vi "Query Error.vi"(8 "error in (no error)":errorcluster, 11 "VISA resource name":refnum<visa-resource-name>) -> (0 "error out":errorcluster, 1 "Error Message":string, 2 "Error Code":i32[](array[numeric]), 3 "VISA resource name out":refnum<visa-resource-name>)   [LabVIEW 2023]
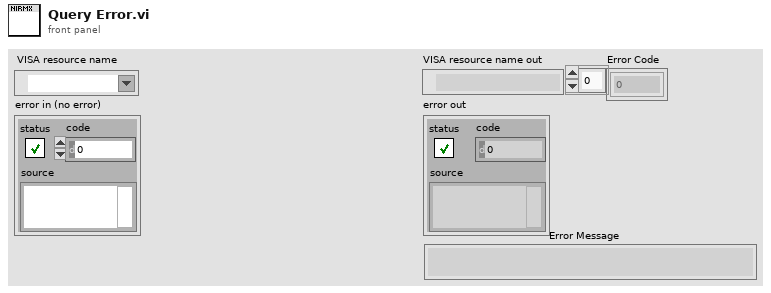
[diagram p1: front panel]
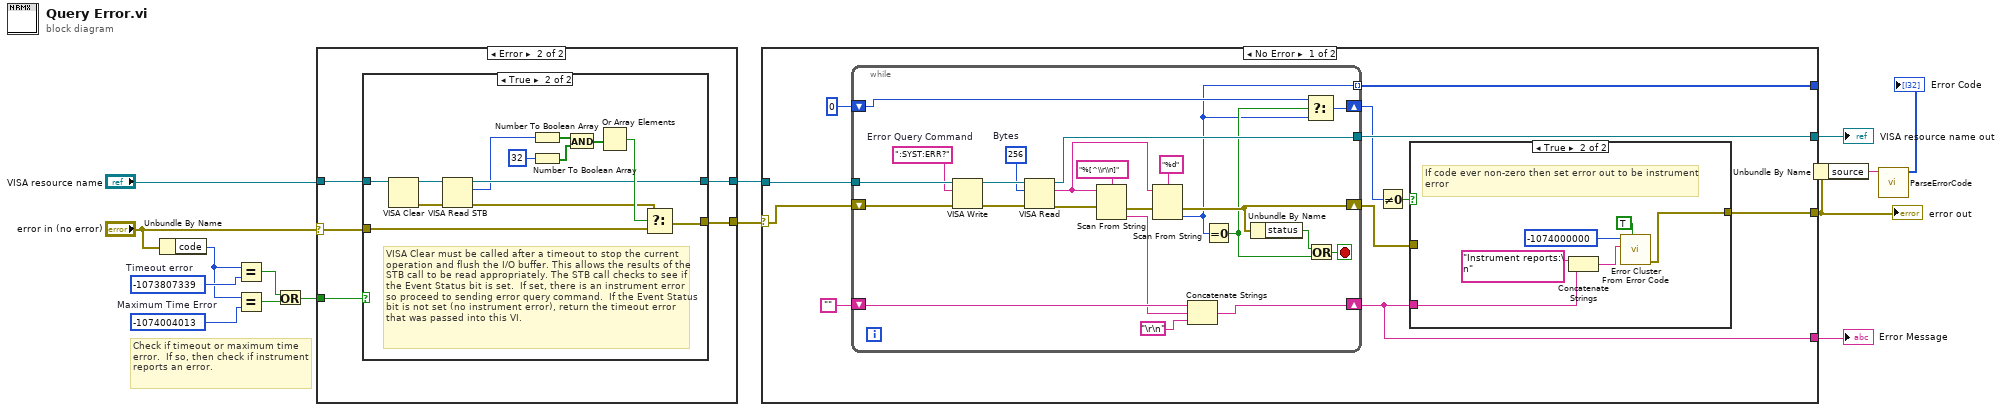
[diagram p0: block diagram]
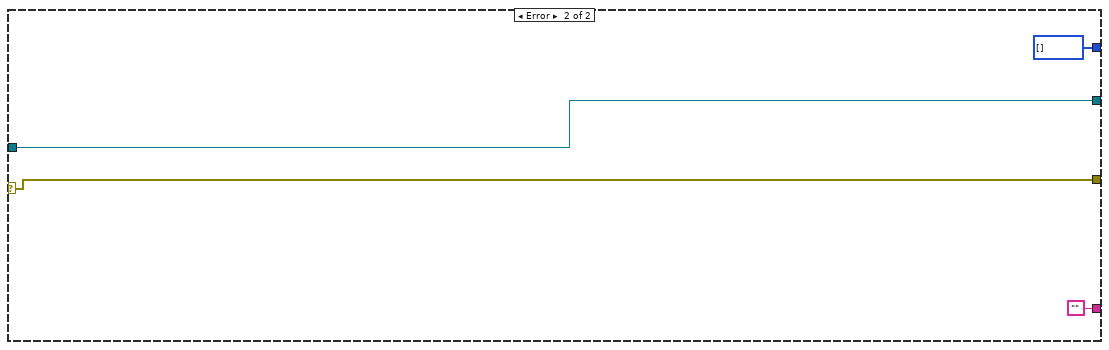
[diagram p5: hidden frame]
diagram:
  w8 = -1074004013  # Maximum Time Error
  w10 = -1073807339  # Timeout error
  # "Check if timeout or maximum time error.  If so, then check if instrument reports an error."
  n1 = Unbundle By Name("error in (no error)") -> ("code"=w9:i32)
  n2 = Equal?(x=w9, y=w10) -> (x = y?=w6:bool)
  n3 = Equal?(x=w9, y=w8) -> (x = y?=w7:bool)
  n4 = Or(x=w6, y=w7) -> (x .or. y?=w5:bool)
  n5 = case shown="Error" "error in (no error)" {
    selector: "error in (no error)" -> [w16 w20]
    tunnel: "VISA resource name" -> [w17 w22]
    tunnel: [w17 w21] -> w12
    tunnel: [w16 w19] -> w13
    tunnel: w5 -> [_ w18]
    frame No Error {
    }
    frame Error {
      n6 = case shown="True" w18 {
        tunnel: w22 -> [w24 w30]
        tunnel: [w24 w27] -> w21
        tunnel: w20 -> [w23 w33]
        tunnel: [w23 w32] -> w19
        frame False {
          # "Error code not a timeout, so best to pass on to user."
        }
        frame True {
          # "VISA Clear must be called after a timeout to stop the current operation and flush the I/O buffer. This allows the results of the  STB call to be read appropriately. The STB call checks to see if the Event Status bit is set.  If set, there is an instrument error so proceed to sending error query command.  If the Event Status bit is not set (no instrument error), return the timeout error that was passed into this VI."
          n7 = VISA Clear(VISA resource name=w30) -> (VISA resource name out=w29:refnum<visa-resource-name>, error out=w28:errorcluster)  [unwired: 1 in]
          n8 = VISA Read STB(8:w28, 11:w29) -> (0:w26:errorcluster, 2:w25:u16, 3:w27:refnum<visa-resource-name>)
          n9 = Number To Boolean Array(number=w25) -> (Boolean array=w34:bool[])
          n10 = Number To Boolean Array(number=32) -> (Boolean array=w36:bool[])
          n11 = And(x=w34, y=w36) -> (x .and. y?=w35:bool[])
          n12 = Or Array Elements(Boolean array=w35) -> (logical OR=w31:bool)
          n13 = Select(t=w26, s=w31, f=w33) -> (s? t:f=w32:errorcluster)
        }
      }
    }
  }
  n14 = case shown="No Error" w13 {
    selector: w13 -> [w39 w79]
    tunnel: [w48 w82] -> w15
    tunnel: w12 -> [w47 w82]
    tunnel: [w38 w79] -> w3
    tunnel: [w42 ""] -> w14
    tunnel: [w41 i32[] []] -> _
    frame No Error {
      n15 = while {
        tunnel: [w78] -> w48
        tunnel: w47 -> [w77]
        shift-right: [w65] -> w42
        shift-left: "" -> [w68]
        shift-right: [w63] -> w43
        shift-left: 0 -> [w64]
        shift-right: [w61] -> w40
        shift-left: w39 -> [w62]
        tunnel: [w56] -> w41 mode=indexing
        stop <- w71 stop-if-true
        w75 = u32 256  # Bytes
        w73 = ":SYST:ERR?"  # Error Query Command
        n16 = VISA Write(VISA resource name=w77, write buffer=w73, error in (no error)=w62) -> (VISA resource name out=w76:refnum<visa-resource-name>, error out=w74:errorcluster)  [unwired: 1 out]
        n17 = VISA Read(VISA resource name=w76, byte count=w75, error in (no error)=w74) -> (VISA resource name out=w78:refnum<visa-resource-name>, read buffer=w69:string, error out=w60:errorcluster)  [unwired: 1 out]
        n18 = Scan From String(format string="%[^\\r\\n]", input string=w69, error in=w60) -> (error out=w59:errorcluster, output 1=w66:string)  [unwired: 2 in, 2 out]
        n19 = Scan From String(format string="%d", input string=w69, error in=w59) -> (error out=w61:errorcluster, output 1=w56:i32)  [unwired: 2 in, 2 out]
        n20 = Concatenate Strings(w68, w66, "\r\n") -> (w65:string)
        n21 = Equal To 0?(x=w56) -> (x = 0?=w57:bool)
        n22 = Unbundle By Name(w61) -> ("status"=w58:bool)
        n23 = Select(t=w64, s=w57, f=w56) -> (s? t:f=w63:i32)
        n24 = Or(x=w58, y=w57) -> (x .or. y?=w71:bool)
      }
      n25 = Not Equal To 0?(x=w43) -> (x != 0?=w44:bool)
      n26 = case shown="True" w44 {
        tunnel: w42 -> [_ w54]
        tunnel: [w49 w50] -> w38
        tunnel: w40 -> [w49 _]
        frame False {
        }
        frame True {
          # "If code ever non-zero then set error out to be instrument error"
          n27 = Concatenate Strings("Instrument reports:\n" ("Source"), w54) -> (w51:string)
          n28 = call <vilib>:"Error Cluster From Error Code.vi"("show call chain? (False)"=TRUE, "error message (\"\")"=w51, "error code (0)"=-1074000000 ("Code")) -> ("error out"=w50:errorcluster)  [unwired: 6 in]
        }
      }
    }
    frame Error {
    }
  }
  "VISA resource name out" <- w15
  "error out" <- w3
  "Error Message" <- w14
  n29 = Unbundle By Name(w3) -> ("source"=w2:string)
  n30 = call "ParseErrorCode.vi"("String"=w2) -> ("number"=→"Error Code":i32[])  [unwired: 10 in]
